vi "AutoCargoShip.vi"(9 "Type":string, 10 "RightSideOfField?":bool, 11 "Coordinates":dbl[](array[numeric])) -> ()   [LabVIEW 2018]
uses:
  Globals.vi
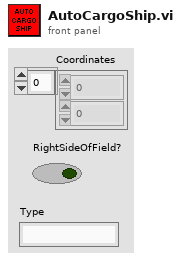
[diagram p1: front panel]
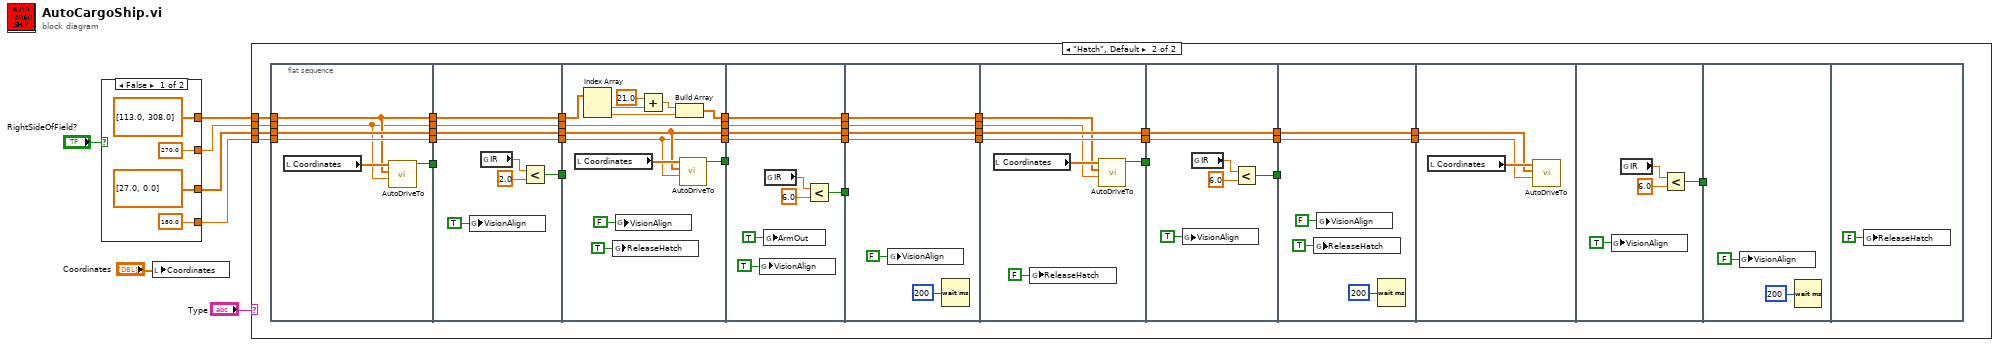
[diagram p0: block diagram]
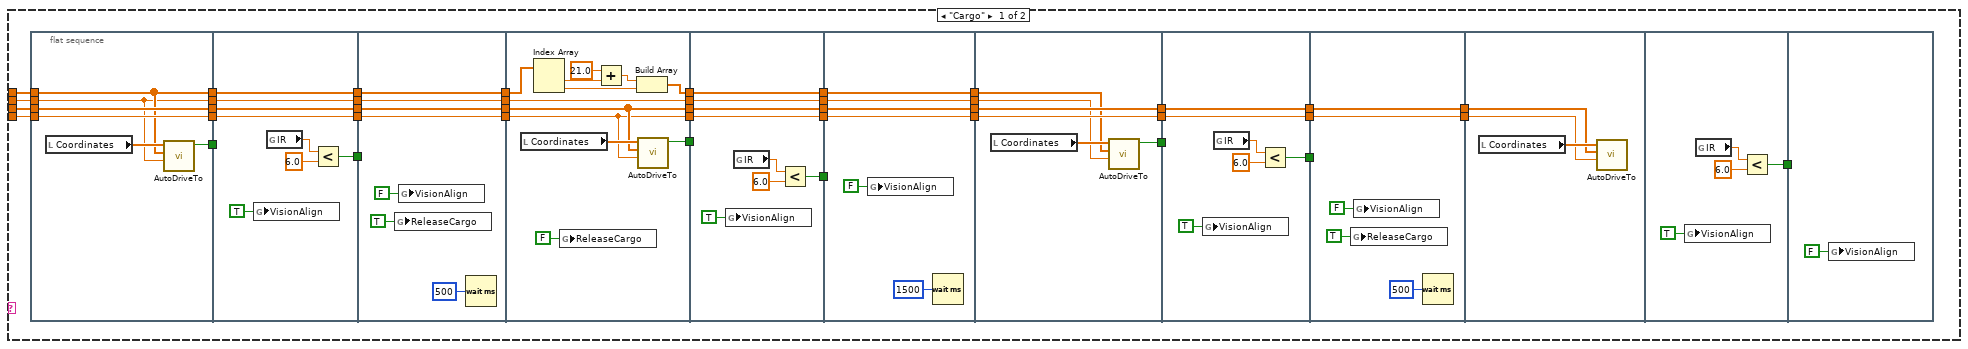
[diagram p2: hidden frame]
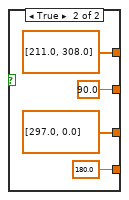
[diagram p3: hidden frame]
diagram:
  n1 = case shown="False" "RightSideOfField?" {
    tunnel: [dbl[] [27.0, 0.0] dbl[] [297.0, 0.0]] -> w5
    tunnel: [270.0 90.0] -> w6
    tunnel: [dbl[] [113.0, 308.0] dbl[] [211.0, 308.0]] -> w2
    tunnel: [180.0 180.0] -> w4
    frame False {
    }
    frame True {
    }
  }
  n2 = local write "Coordinates"("Coordinates") -> ()
  n3 = case shown="\"Hatch\", Default" "Type" {
    tunnel: w6 -> [w18 w132]
    tunnel: w5 -> [w17 w131]
    tunnel: w4 -> [w16 w130]
    tunnel: w2 -> [w19 w129]
    frame "Cargo" {
      n4 = flat-sequence {
        tunnel: [w62] -> w56
        tunnel: w19 -> [w58]
        tunnel: w18 -> [w57]
        tunnel: w17 -> [w61]
        tunnel: w16 -> [w60]
        tunnel: [w61] -> w55
        tunnel: [w60] -> w54
        tunnel: [w58] -> w53
        tunnel: [w57] -> w52
        tunnel: [w67] -> w51
        tunnel: w56 -> [_]
        tunnel: w55 -> [w66]
        tunnel: w54 -> [w65]
        tunnel: [w66] -> w50
        tunnel: [w65] -> w49
        tunnel: [w64] -> w48
        tunnel: w53 -> [w64]
        tunnel: w52 -> [w63]
        tunnel: [w63] -> w47
        tunnel: w51 -> [_]
        tunnel: w50 -> [w77]
        tunnel: [w77] -> w46
        tunnel: w49 -> [w76]
        tunnel: [w76] -> w45
        tunnel: w48 -> [w75]
        tunnel: [w75] -> w44
        tunnel: w47 -> [w74]
        tunnel: [w74] -> w43
        tunnel: w46 -> [w86]
        tunnel: w45 -> [w85]
        tunnel: [w88] -> w42
        tunnel: [w78] -> w41
        tunnel: w44 -> [w79]
        tunnel: w43 -> [w87]
        tunnel: [w87] -> w40
        tunnel: [w86] -> w39
        tunnel: [w85] -> w38
        tunnel: w42 -> [_]
        tunnel: w41 -> [w97]
        tunnel: [w97] -> w37
        tunnel: w40 -> [w96]
        tunnel: [w96] -> w36
        tunnel: w39 -> [w95]
        tunnel: [w95] -> w35
        tunnel: w38 -> [w94]
        tunnel: [w94] -> w34
        tunnel: [w91] -> w33
        tunnel: [w103] -> w32
        tunnel: w37 -> [w103]
        tunnel: [w102] -> w31
        tunnel: w36 -> [w102]
        tunnel: [w101] -> w30
        tunnel: w35 -> [w101]
        tunnel: [w100] -> w29
        tunnel: w34 -> [w100]
        tunnel: w33 -> [_]
        tunnel: w32 -> [w106]
        tunnel: w31 -> [w105]
        tunnel: w30 -> [w109]
        tunnel: w29 -> [w108]
        tunnel: [w109] -> w28
        tunnel: [w108] -> w27
        tunnel: [w104] -> w26
        tunnel: w28 -> [w115]
        tunnel: w27 -> [w114]
        tunnel: [w115] -> w25
        tunnel: [w114] -> w24
        tunnel: [w110] -> w23
        tunnel: w26 -> [_]
        tunnel: w25 -> [w120]
        tunnel: w24 -> [w119]
        tunnel: w23 -> [_]
        tunnel: [w120] -> w22
        tunnel: [w119] -> w21
        tunnel: w22 -> [w122]
        tunnel: w21 -> [w121]
        tunnel: [w124] -> w20
        tunnel: w20 -> [_]
        frame #0 {
          n5 = local read "Coordinates"() -> (w59:dbl[])
          n6 = call "AutoDriveTo.vi"("EndAngle"=w57, "EndCoordinates"=w58, "Coordinates"=w59) -> ("ThereYet?"=w62:bool)  [unwired: 8 in]
        }
        frame #1 {
          n7 = global write "Globals.vi" "VisionAlign"(TRUE ("VisionAlign")) -> ()
          n8 = global read "Globals.vi" "IR"() -> (w69:dbl)
          n9 = Less?(x=w69, y=6.0) -> (x < y?=w67:bool)
        }
        frame #2 {
          n10 = global write "Globals.vi" "ReleaseCargo"(TRUE ("ReleaseCargo")) -> ()
          n11 = global write "Globals.vi" "VisionAlign"(FALSE ("VisionAlign")) -> ()
          n12 = Wait (ms)(milliseconds to wait=u32 500) -> ()  [unwired: 1 out]
        }
        frame #3 {
          n13 = local read "Coordinates"() -> (w89:dbl[])
          n14 = Index Array(array=w79) -> (element #1=w81:dbl, element #2=w83:dbl)  [unwired: 2 in]
          n15 = global write "Globals.vi" "ReleaseCargo"(FALSE ("ReleaseCargo")) -> ()
          n16 = Add(x=21.0, y=w81) -> (x+y=w82:dbl)
          n17 = Build Array(w82, w83) -> (w78:dbl[])
          n18 = call "AutoDriveTo.vi"("EndAngle"=w85, "EndCoordinates"=w86, "Coordinates"=w89) -> ("ThereYet?"=w88:bool)  [unwired: 8 in]
        }
        frame #4 {
          n19 = global write "Globals.vi" "VisionAlign"(TRUE ("VisionAlign")) -> ()
          n20 = global read "Globals.vi" "IR"() -> (w93:dbl)
          n21 = Less?(x=w93, y=6.0) -> (x < y?=w91:bool)
        }
        frame #5 {
          n22 = global write "Globals.vi" "VisionAlign"(FALSE ("VisionAlign")) -> ()
          n23 = Wait (ms)(milliseconds to wait=u32 1500) -> ()  [unwired: 1 out]
        }
        frame #6 {
          n24 = local read "Coordinates"() -> (w107:dbl[])
          n25 = call "AutoDriveTo.vi"("EndAngle"=w105, "EndCoordinates"=w106, "Coordinates"=w107) -> ("ThereYet?"=w104:bool)  [unwired: 8 in]
        }
        frame #7 {
          n26 = global write "Globals.vi" "VisionAlign"(TRUE ("VisionAlign")) -> ()
          n27 = global read "Globals.vi" "IR"() -> (w112:dbl)
          n28 = Less?(x=w112, y=6.0) -> (x < y?=w110:bool)
        }
        frame #8 {
          n29 = global write "Globals.vi" "ReleaseCargo"(TRUE ("ReleaseHatch")) -> ()
          n30 = global write "Globals.vi" "VisionAlign"(FALSE ("VisionAlign")) -> ()
          n31 = Wait (ms)(milliseconds to wait=u32 500) -> ()  [unwired: 1 out]
        }
        frame #9 {
          n32 = local read "Coordinates"() -> (w123:dbl[])
          n33 = call "AutoDriveTo.vi"("EndAngle"=w121, "EndCoordinates"=w122, "Coordinates"=w123) -> ()  [unwired: 8 in, 1 out]
        }
        frame #10 {
          n34 = global write "Globals.vi" "VisionAlign"(TRUE ("VisionAlign")) -> ()
          n35 = global read "Globals.vi" "IR"() -> (w126:dbl)
          n36 = Less?(x=w126, y=6.0) -> (x < y?=w124:bool)
        }
        frame #11 {
          n37 = global write "Globals.vi" "VisionAlign"(FALSE ("VisionAlign")) -> ()
        }
      }
    }
    frame "Hatch", Default {
      n38 = flat-sequence {
        tunnel: [w171] -> w165
        tunnel: w129 -> [w167]
        tunnel: w132 -> [w166]
        tunnel: w131 -> [w170]
        tunnel: w130 -> [w169]
        tunnel: [w170] -> w164
        tunnel: [w169] -> w163
        tunnel: [w167] -> w162
        tunnel: [w166] -> w161
        tunnel: [w176] -> w160
        tunnel: w165 -> [_]
        tunnel: w164 -> [w175]
        tunnel: w163 -> [w174]
        tunnel: [w175] -> w159
        tunnel: [w174] -> w158
        tunnel: [w172] -> w157
        tunnel: w162 -> [w172]
        tunnel: w161 -> [w173]
        tunnel: [w173] -> w156
        tunnel: w160 -> [_]
        tunnel: w159 -> [w189]
        tunnel: w158 -> [w188]
        tunnel: [w191] -> w155
        tunnel: [w180] -> w154
        tunnel: w157 -> [w183]
        tunnel: w156 -> [w190]
        tunnel: [w190] -> w153
        tunnel: [w189] -> w152
        tunnel: [w188] -> w151
        tunnel: w155 -> [_]
        tunnel: w154 -> [w201]
        tunnel: [w201] -> w150
        tunnel: w153 -> [w200]
        tunnel: [w200] -> w149
        tunnel: w152 -> [w199]
        tunnel: [w199] -> w148
        tunnel: w151 -> [w198]
        tunnel: [w198] -> w147
        tunnel: [w195] -> w146
        tunnel: [w207] -> w145
        tunnel: w150 -> [w207]
        tunnel: [w206] -> w144
        tunnel: w149 -> [w206]
        tunnel: [w205] -> w143
        tunnel: w148 -> [w205]
        tunnel: [w204] -> w142
        tunnel: w147 -> [w204]
        tunnel: w146 -> [_]
        tunnel: w145 -> [w210]
        tunnel: w144 -> [w209]
        tunnel: w143 -> [w214]
        tunnel: w142 -> [w213]
        tunnel: [w214] -> w141
        tunnel: [w213] -> w140
        tunnel: [w208] -> w139
        tunnel: w141 -> [w220]
        tunnel: w140 -> [w219]
        tunnel: [w220] -> w138
        tunnel: [w219] -> w137
        tunnel: [w215] -> w136
        tunnel: w139 -> [_]
        tunnel: w138 -> [w225]
        tunnel: w137 -> [w224]
        tunnel: w136 -> [_]
        tunnel: [w225] -> w135
        tunnel: [w224] -> w134
        tunnel: w135 -> [w227]
        tunnel: w134 -> [w226]
        tunnel: [w229] -> w133
        tunnel: w133 -> [_]
        frame #0 {
          n39 = local read "Coordinates"() -> (w168:dbl[])
          n40 = call "AutoDriveTo.vi"("EndAngle"=w166, "EndCoordinates"=w167, "Coordinates"=w168) -> ("ThereYet?"=w171:bool)  [unwired: 8 in]
        }
        frame #1 {
          n41 = global write "Globals.vi" "VisionAlign"(TRUE ("VisionAlign")) -> ()
          n42 = global read "Globals.vi" "IR"() -> (w178:dbl)
          n43 = Less?(x=w178, y=2.0) -> (x < y?=w176:bool)
        }
        frame #2 {
          n44 = local read "Coordinates"() -> (w192:dbl[])
          n45 = Index Array(array=w183) -> (element #1=w185:dbl, element #2=w181:dbl)  [unwired: 2 in]
          n46 = global write "Globals.vi" "ReleaseHatch"(TRUE ("ReleaseHatch")) -> ()
          n47 = global write "Globals.vi" "VisionAlign"(FALSE ("VisionAlign")) -> ()
          n48 = Add(x=21.0, y=w185) -> (x+y=w182:dbl)
          n49 = Build Array(w182, w181) -> (w180:dbl[])
          n50 = call "AutoDriveTo.vi"("EndAngle"=w188, "EndCoordinates"=w189, "Coordinates"=w192) -> ("ThereYet?"=w191:bool)  [unwired: 8 in]
        }
        frame #3 {
          n51 = global write "Globals.vi" "VisionAlign"(TRUE ("VisionAlign")) -> ()
          n52 = global write "Globals.vi" "ArmOut"(TRUE ("ArmOut")) -> ()
          n53 = global read "Globals.vi" "IR"() -> (w197:dbl)
          n54 = Less?(x=w197, y=6.0) -> (x < y?=w195:bool)
        }
        frame #4 {
          n55 = global write "Globals.vi" "VisionAlign"(FALSE ("VisionAlign")) -> ()
          n56 = Wait (ms)(milliseconds to wait=u32 200) -> ()  [unwired: 1 out]
        }
        frame #5 {
          n57 = local read "Coordinates"() -> (w211:dbl[])
          n58 = global write "Globals.vi" "ReleaseHatch"(FALSE ("ReleaseHatch")) -> ()
          n59 = call "AutoDriveTo.vi"("EndAngle"=w209, "EndCoordinates"=w210, "Coordinates"=w211) -> ("ThereYet?"=w208:bool)  [unwired: 8 in]
        }
        frame #6 {
          n60 = global write "Globals.vi" "VisionAlign"(TRUE ("VisionAlign")) -> ()
          n61 = global read "Globals.vi" "IR"() -> (w217:dbl)
          n62 = Less?(x=w217, y=6.0) -> (x < y?=w215:bool)
        }
        frame #7 {
          n63 = global write "Globals.vi" "ReleaseHatch"(TRUE ("ReleaseHatch")) -> ()
          n64 = global write "Globals.vi" "VisionAlign"(FALSE ("VisionAlign")) -> ()
          n65 = Wait (ms)(milliseconds to wait=u32 200) -> ()  [unwired: 1 out]
        }
        frame #8 {
          n66 = local read "Coordinates"() -> (w228:dbl[])
          n67 = call "AutoDriveTo.vi"("EndAngle"=w226, "EndCoordinates"=w227, "Coordinates"=w228) -> ()  [unwired: 8 in, 1 out]
        }
        frame #9 {
          n68 = global write "Globals.vi" "VisionAlign"(TRUE ("VisionAlign")) -> ()
          n69 = global read "Globals.vi" "IR"() -> (w231:dbl)
          n70 = Less?(x=w231, y=6.0) -> (x < y?=w229:bool)
        }
        frame #10 {
          n71 = global write "Globals.vi" "VisionAlign"(FALSE ("VisionAlign")) -> ()
          n72 = Wait (ms)(milliseconds to wait=u32 200) -> ()  [unwired: 1 out]
        }
        frame #11 {
          n73 = global write "Globals.vi" "ReleaseHatch"(FALSE ("ReleaseHatch")) -> ()
        }
      }
    }
  }
